vi "List Words in String.vi"(11 "String":string) -> (3 "Array":T1[](array[typedef]))   [LabVIEW 2020, in "Words to Numbers Converter.lvclass"]
uses:
  Words to Numbers Converter.lvclass
  Word in String.ctl
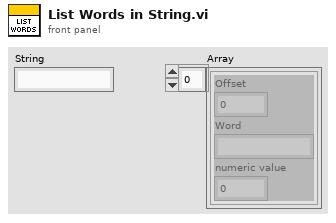
[diagram p1: front panel]
types:
  T1 = typedef "Words to Numbers Converter.lvclass/Word in String.ctl" = cluster{"Offset":i32, "Word":string, "numeric value":i32}
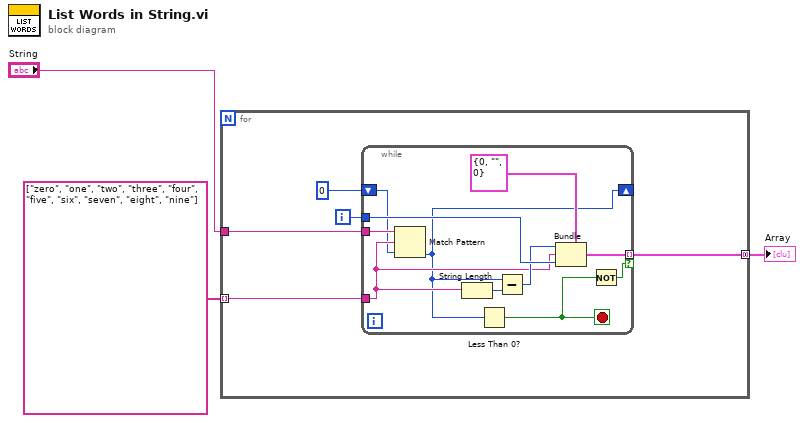
[diagram p0: block diagram]
diagram:
  n1 = for {
    tunnel: string[] ["zero", "one", "two", "three", "four", "five", "six", "seven", "eight", "nine"] -> [w8] mode=indexing
    tunnel: [w6] -> w1 mode=concatenating
    tunnel: "String" -> [w5]
    i -> [w7]
    n2 = while {
      tunnel: w8 -> [w14]
      tunnel: w7 -> [w19]
      tunnel: [w18] -> w6 mode=indexing if=w16
      tunnel: w5 -> [w11]
      shift-right: [w9] -> _
      shift-left: 0 ("offset (0)") -> [w10]
      stop <- w17 stop-if-true
      n3 = Match Pattern(string=w11, regular expression=w14, offset (0)=w10) -> (offset past match=w9:i32)  [unwired: 3 out]
      n4 = String Length(string=w14) -> (length=w13:i32)
      n5 = Less Than 0?(x=w9) -> (x < 0?=w17:bool)
      n6 = Subtract(x=w9, y=w13) -> (x-y=w15:i32)
      n7 = Bundle(cluster=T1 {"Offset"=0, "Word"="", "numeric value"=0} ("Cluster"), "Offset"=w15, "Word"=w14, "numeric value"=w19) -> (w18:T1)
      n8 = Not(x=w17) -> (.not. x?=w16:bool)
    }
  }
  "Array" <- w1
